vi "Averaging.vi"(3 "address":string="10.0.0.98") -> (1 "output cluster":cluster{dbl[], dbl[]}(graph))   [LabVIEW 2009]
uses:
  <vilib>/Analysis/NI_AALBase.lvlib
panel:
  out "Numeric":i32
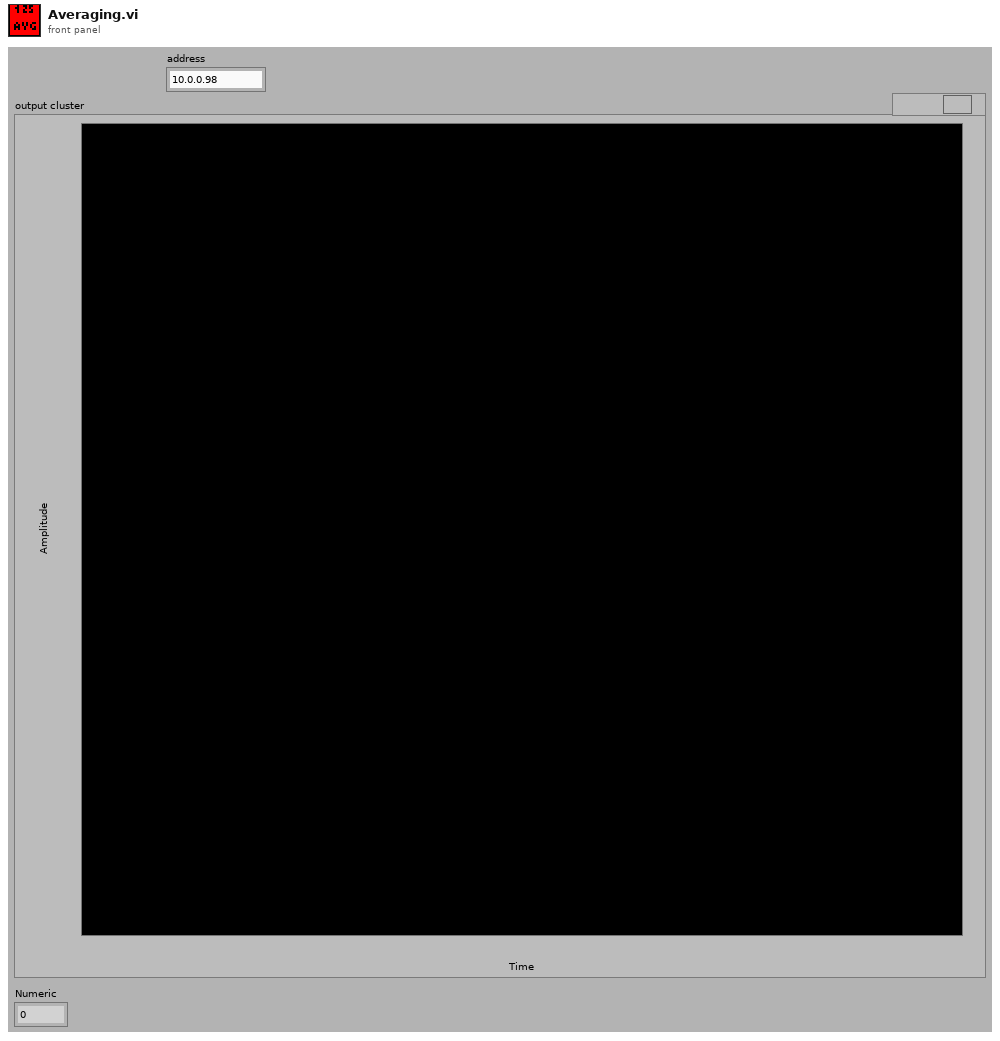
[diagram p1: front panel]
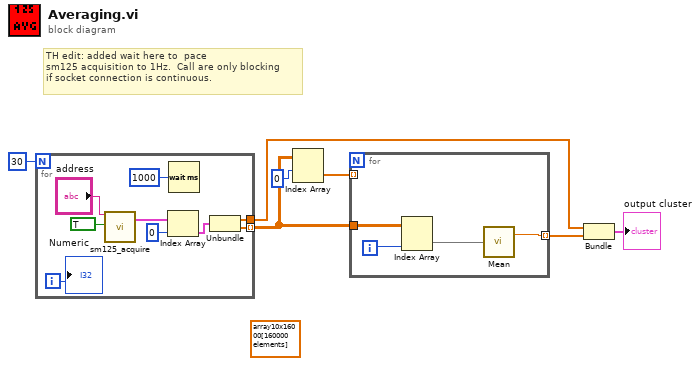
[diagram p0: block diagram]
diagram:
  (unwired) dbl[][] array10x16000[160000 elements] ("Array")
  # "TH edit: added wait here to  pace\nsm125 acquisition to 1Hz.  Call are only blocking\nif socket connection is continuous."
  n1 = for {
    N: 30 -> [_]
    tunnel: [w12] -> w4 mode=indexing
    tunnel: [w11] -> w2
    i -> [w9]
    n2 = call "sm125_acquire.vi"("address"="address", "open and close"=TRUE) -> ("Output graph"=w14:cluster{dbl[], dbl[]}[])  [unwired: 14 in, 3 out]
    n3 = Index Array(array=w14, index=0) -> (element=w13:cluster{dbl[], dbl[]})
    n4 = Wait (ms)(milliseconds to wait=u32 1000) -> ()  [unwired: 1 out]
    n5 = Unbundle(w13) -> (w11:dbl[], w12:dbl[])
    "Numeric" <- w9
  }
  n6 = Index Array(array=w4, index (row)=0 ("disabled index (col)")) -> (element=w7:dbl[])  [unwired: 1 in]
  n7 = for {
    tunnel: w4 -> [w19]
    tunnel: w7 -> [_] mode=indexing
    tunnel: [w17] -> w3 mode=indexing
    i -> [w20]
    n8 = Index Array(array=w19, index (col)=w20) -> (element=w18:dbl[])  [unwired: 1 in]
    n9 = call <vilib>:"Mean.vi"("X"=w18) -> ("mean"=w17:dbl)  [unwired: 1 out]
  }
  n10 = Bundle(w2, w3) -> (→"output cluster":cluster{dbl[], dbl[]})  [unwired: 1 in]
